vi "DISH ERD List.vi"(8 "Error In":errorcluster, 11 "Disable ERD (Main)":bool) -> (0 "Error Out":errorcluster, 1 "GEA Inputs":T1 {"Destination" format="%.0x"; "Source" format="%.0x"}, 2 "Array":string[](array[string]), 3 "Read ERD List":T2[](array[typedef]) {"ERD Number" format="%.0x"})   [LabVIEW 2016]
uses:
  type defs/ERD Read Data In.ctl
  type defs/Data Type.ctl
  type defs/Source_Destination.ctl
  <vilib>/Utility/error.llb/whitespace.ctl
  library/GEA2_Toolkit.lvlib
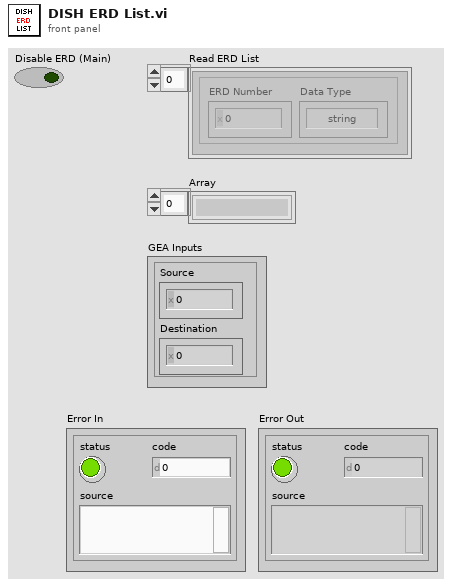
[diagram p1: front panel]
types:
  T1 = typedef "GEA2_Toolkit.lvlib/Source_Destination.ctl" = cluster{"Source":u8, "Destination":u8}
  T2 = typedef "GEA2_Toolkit.lvlib/ERD Read Data In.ctl" = cluster{"ERD Number":u16, "Data Type":T3}
  T3 = typedef "GEA2_Toolkit.lvlib/Data Type.ctl" = enum16{"string", "boolean", "uint8_t", "uint16_t", "uint32_t", "uint64_t"}
  T4 = typedef "whitespace.ctl" = u16
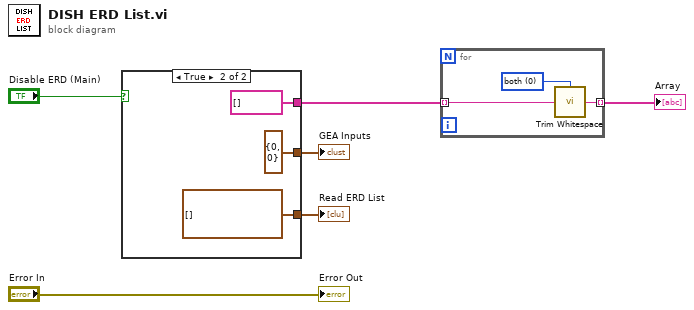
[diagram p0: block diagram]
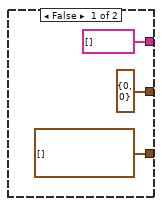
[diagram p2: hidden frame]
diagram:
  n1 = case shown="True" "Disable ERD (Main)" {
    tunnel: [T1 {"Source"=0, "Destination"=0} ("GEA Inputs") T1 {"Source"=0, "Destination"=0} ("GEA Inputs")] -> w4
    tunnel: [string[] [] string[] []] -> w2
    tunnel: [T2[] [] ("Read ERD List") T2[] [] ("Read ERD List")] -> w5
    frame False {
    }
    frame True {
    }
  }
  "Read ERD List" <- w5
  "GEA Inputs" <- w4
  n2 = for {
    tunnel: w2 -> [w14] mode=indexing
    tunnel: [w13] -> w1 mode=indexing
    w15 = T4 0 items=["both", "start of string", "end of string"] ("location (both)")
    n3 = call <vilib>:"Trim Whitespace.vi"("string"=w14, "location (both)"=w15) -> ("trimmed string"=w13:string)
  }
  "Array" <- w1
  "Error Out" <- "Error In"
